vi "Eigenvalues and Vectors.vi"   [LabVIEW 2020, in "NI_AALPro.lvlib"]
doc: "Finds the eigenvalues and right eigenvectors of the square <B>Input Matrix</B>. Wire data to the <B>Input Matrix</B> input to determine the polymorphic instance to use or manually select the instance."
uses:
  <vilib>/Analysis/NI_AALPro.lvlib
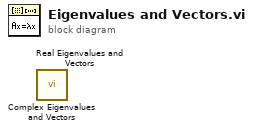
[diagram p0: block diagram]
diagram:
  n1 = call <vilib>:"Complex Eigenvalues and Vectors.vi"() -> ()  [unwired: 3 in, 3 out]
  n2 = call <vilib>:"Real Eigenvalues and Vectors.vi"() -> ()  [unwired: 3 in, 3 out]
